vi "ToString.vi"(0 "reference in":refnum<class "Gear.lvclass">, 5 "error in (no error)":errorcluster) -> (14 "reference out":refnum<class "Gear.lvclass">, 15 "string":string, 19 "error out":errorcluster)   [LabVIEW 2013, in "Gear.lvclass"]
doc: "Defines a method that allows a class to return one string as a representation of the object."
uses:
  Gear.lvclass
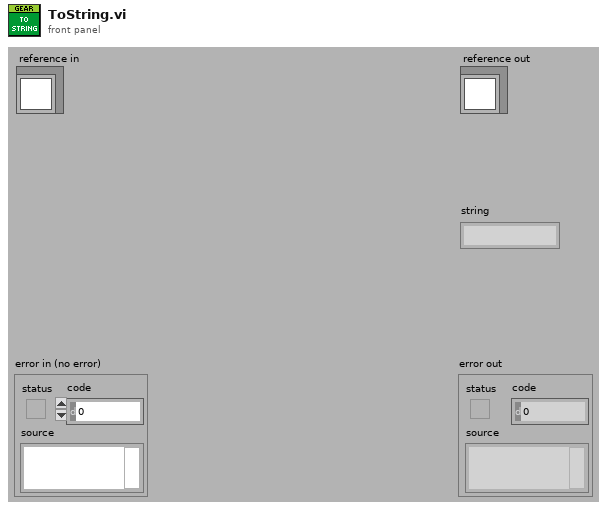
[diagram p1: front panel]
types:
  T1 = typedef "Gear.lvclass/ObjectAttributes.ctl" = cluster{"MyAttribute":dbl}
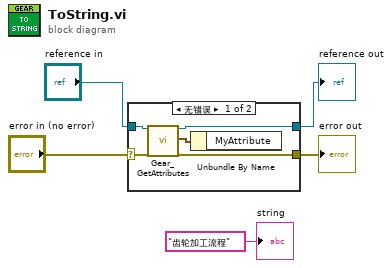
[diagram p0: block diagram]
diagram:
  n1 = case shown="无错误" "error in (no error)" {
    selector: "error in (no error)" -> [w10 w12]
    tunnel: [w9 w12] -> w4
    tunnel: [w8 w11] -> w2
    tunnel: "reference in" -> [w6 w11]
    frame No Error {
      n2 = call "Gear_GetAttributes.vi"("reference in"=w6, "error in (no error)"=w10) -> ("reference out"=w8:refnum<class "Gear.lvclass">, "attributes"=w7:T1, "error out"=w9:errorcluster)  [unwired: 14 in, 1 out]
      n3 = Unbundle By Name(w7) -> ()  [unwired: 1 out]
    }
    frame Error {
    }
  }
  "error out" <- w4
  "reference out" <- w2
  "string" <- "齿轮加工流程" ("string")
